vi "FID mit Propan Linearisieren.vi"(10 "Werte":string[](array[string])) -> (2 "Werte":string[](array[string]))   [LabVIEW 2015]
uses:
  ABB Kalibrieren/Komm AO2000/Aktionen FID Kal Komponente.ctl
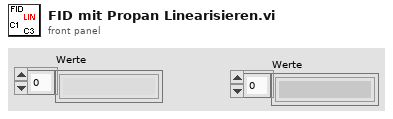
[diagram p1: front panel]
types:
  T1 = typedef "ABB Kalibrieren.lvlib/EL3000.lvlib/Aktionen FID Kal Komponente.ctl" = enum16{"lesen", "setzen", "laden", "speichern", "Lin"}
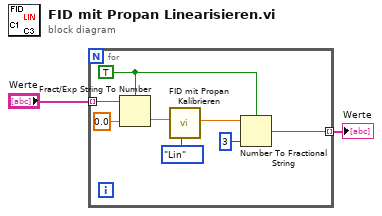
[diagram p0: block diagram]
diagram:
  n1 = for {
    tunnel: "Werte" -> [w10] mode=indexing
    tunnel: [w3] -> w1 mode=indexing
    w4 = TRUE ("Systemdezimalzeichen verwenden (T)")
    n2 = Fract/Exp String To Number(use system decimal point (T)=w4, string=w10, default (0 dbl)=sgl 0.0 ("Standard (0 DBL)")) -> (number=w8:sgl)  [unwired: 1 in, 1 out]
    n3 = call "FID mit Propan Kalibrieren.vi"("Aktionen"=Aktionen_FID_Kal_Komponente."Lin", "Wert"=w8) -> ("Wert"=w6:sgl)  [unwired: 8 in, 1 out]
    n4 = Number To Fractional String(use system decimal point (T)=w4, number=w6, precision (6)=i16 3 ("Genauigkeit (6)")) -> (F-format string=w3:string)  [unwired: 1 in]
  }
  "Werte" <- w1
